vi "MainPicFloatMotV1PIC.vi"() -> ()   [LabVIEW 2010]
uses:
  <vilib>/Instr/_visa.llb/VISA Flush IO Buffer Mask.ctl
  Variable globale 1.vi
  <vilib>/Instr/_visa.llb/VISA Configure Serial Port (Instr).vi
panel:
  out "tableau inversé 2":u8[](array[numeric])
  out "tableau inversé":i8[](array[numeric])
  out "error out 2":errorcluster caption="sortie d'erreur"
  in  "Type":i32=139 min=138 max=139
  out "Float recu":sgl
  in  "Float envoyé":sgl=25.45
  out "Iteration 3":i32
  out "Iteration reception":i32
  out "Iteration Envoi":i32
  out "Checksum calculé":i32
  out "Checksum reçu":i32
  out "Type de donnee (ID)":i32
  out "Byte Start ?":bool
  out "Retour 2":string
  in  "stop secu":bool
  in  "STOP":bool
  out "error out":errorcluster caption="sortie d'erreur"
  in  "baud rate (9600)":u32=9600 caption="débit en bauds (9600)"
  in  "Port Com":refnum<visa-resource-name>="COM7" caption="Nom de ressource VISA"
  # "Envoi"
  # "Réception"
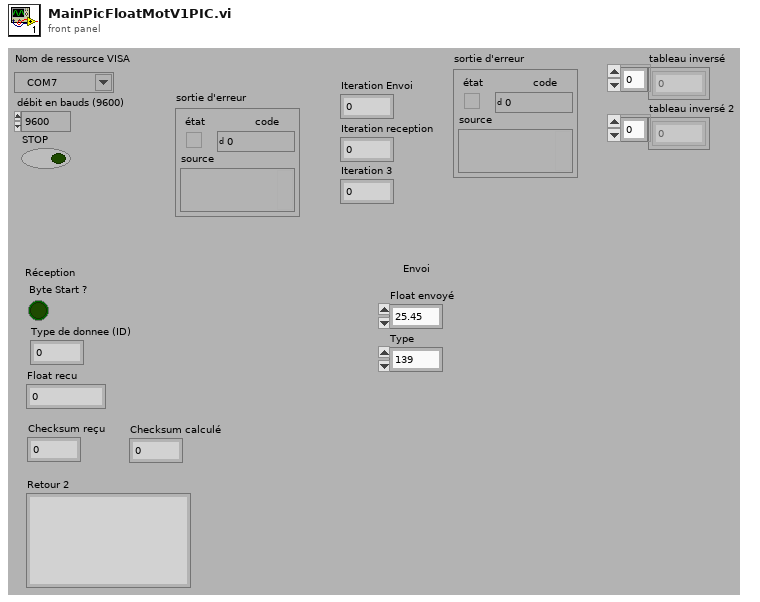
[diagram p1: front panel]
types:
  T1 = typedef "VISA Flush IO Buffer Mask.ctl" = u16
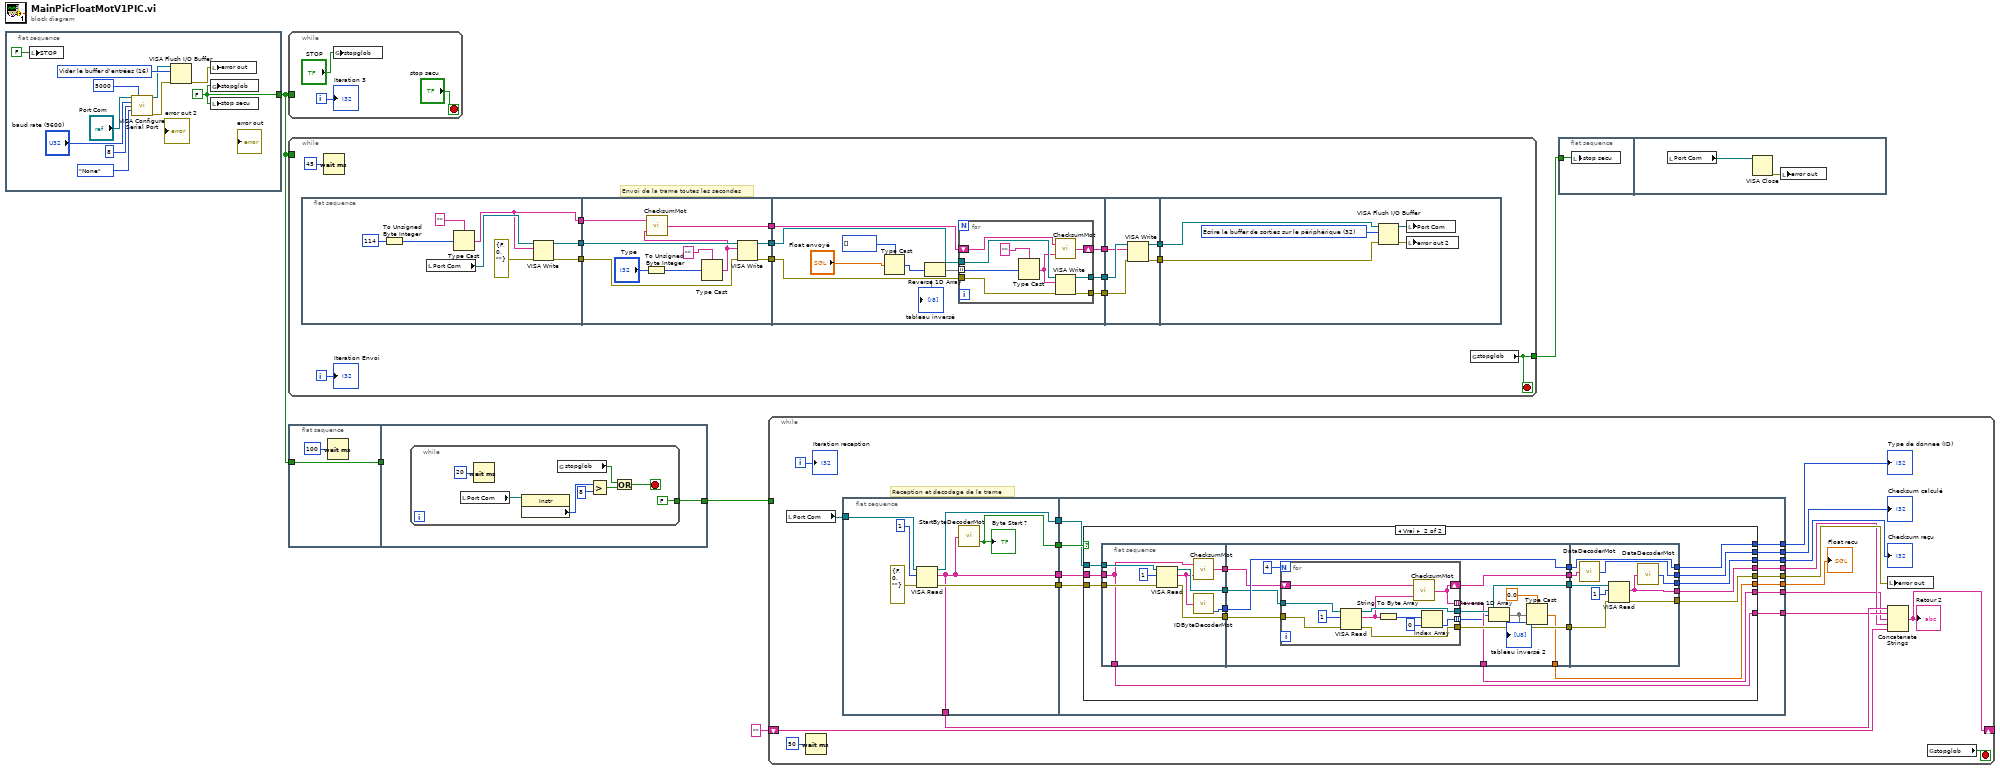
[diagram p0: block diagram]
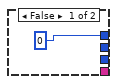
[diagram p2: hidden frame]
diagram:
  n1 = flat-sequence {
    tunnel: [w8] -> w3
    frame #0 {
      w8 = FALSE
      w11 = T1 16 items=["Vider le buffer d'entrées"=16, "Écrire le buffer de sorties sur le périphérique"=32, "Vider le buffer d'entrées (Pas d'E/S)"=64, "Vider le buffer de sorties"=128] ("Mask")
      n2 = local write "STOP"(FALSE) -> ()
      n3 = call-poly "VISA Configure Serial Port"("VISA resource name"="Port Com", "timeout (10sec)"=u32 5000, "baud rate (9600)"="baud rate (9600)", "data bits (8)"=u16 8, "parity (0:none)"=enum16{"None", "Odd", "Even", "Mark", "Space"}."None") -> ("VISA resource name out"=w7:refnum<visa-resource-name>, "error out"=w6:errorcluster)  [unwired: 9 in]
      n4 = VISA Flush I/O Buffer(VISA resource name=w7, mask (16)=w11, error in (no error)=w6) -> (error out=w9:errorcluster)  [unwired: 1 out]
      n5 = local write "error out"(w9) -> ()
      n6 = global write "Variable globale 1.vi" "stopglob"(w8) -> ()
      n7 = local write "stop secu"(w8) -> ()
    }
  }
  n8 = while {
    tunnel: w3 -> [_]
    i -> [w17]
    stop <- "stop secu" stop-if-true
    n9 = global write "Variable globale 1.vi" "stopglob"("STOP") -> ()
    "Iteration 3" <- w17
  }
  n10 = while {
    tunnel: [w27] -> w5
    tunnel: w3 -> [_]
    i -> [w26]
    stop <- w27 stop-if-true
    # "Envoi de la trame toutes les secondes"
    n11 = flat-sequence {
      tunnel: [w38] -> w33
      tunnel: [w37] -> w32
      tunnel: [w36] -> w29
      tunnel: w33 -> [w51]
      tunnel: w32 -> [w50]
      tunnel: [w49] -> w31
      tunnel: [w48] -> w30
      tunnel: w29 -> [w47]
      tunnel: [w46] -> w28
      tunnel: w31 -> [w57]
      tunnel: w30 -> [w59]
      tunnel: w28 -> [w55]
      tunnel: [w58] -> w25
      tunnel: [w56] -> w24
      tunnel: [w54] -> w23
      tunnel: w25 -> [w75]
      tunnel: w24 -> [w74]
      tunnel: w23 -> [w73]
      tunnel: [w72] -> w21
      tunnel: [w71] -> w20
      tunnel: w21 -> [w80]
      tunnel: w20 -> [w79]
      frame #0 {
        n12 = To Unsigned Byte Integer(number=114) -> (unsigned 8bit integer=w35:u8)
        n13 = local read "Port Com"() -> (w41:refnum<visa-resource-name>)
        n14 = Type Cast(type="", x=w35) -> (*(type *) &x=w36:string)
        n15 = VISA Write(VISA resource name=w41, write buffer=w36, error in (no error)=errorcluster {"status"=FALSE, "code"=0, "source"=""} ("entrée d'erreur (pas d'erreur)")) -> (VISA resource name out=w38:refnum<visa-resource-name>, error out=w37:errorcluster)  [unwired: 1 out]
      }
      frame #1 {
        n16 = To Unsigned Byte Integer(number="Type") -> (unsigned 8bit integer=w44:u8)
        n17 = Type Cast(type="", x=w44) -> (*(type *) &x=w42:string)
        n18 = call "ChecksumMot.vi"("Byte2"=w42, "Byte1"=w47) -> ("chaîne"=w46:string)
        n19 = VISA Write(VISA resource name=w51, write buffer=w42, error in (no error)=w50) -> (VISA resource name out=w48:refnum<visa-resource-name>, error out=w49:errorcluster)  [unwired: 1 out]
      }
      frame #2 {
        n20 = Type Cast(type=i8[] [] ("tableau d'octets non signés"), x="Float envoyé") -> (*(type *) &x=w53:i8[])
        n21 = Reverse 1D Array(array=w53) -> (reversed array=w52:i8[])
        "tableau inversé" <- w52
        n22 = for {
          tunnel: w52 -> [w70] mode=indexing
          tunnel: w59 -> [w68]
          tunnel: [w67] -> w58
          tunnel: w57 -> [w66]
          tunnel: [w65] -> w56
          shift-right: [w62] -> w54
          shift-left: w55 -> [w64]
          n23 = Type Cast(type="", x=w70) -> (*(type *) &x=w63:string)
          n24 = call "ChecksumMot.vi"("Byte2"=w63, "Byte1"=w64) -> ("chaîne"=w62:string)
          n25 = VISA Write(VISA resource name=w68, write buffer=w63, error in (no error)=w66) -> (VISA resource name out=w67:refnum<visa-resource-name>, error out=w65:errorcluster)  [unwired: 1 out]
        }
      }
      frame #3 {
        n26 = VISA Write(VISA resource name=w75, write buffer=w73, error in (no error)=w74) -> (VISA resource name out=w72:refnum<visa-resource-name>, error out=w71:errorcluster)  [unwired: 1 out]
      }
      frame #4 {
        w76 = T1 32 items=["Vider le buffer d'entrées"=16, "Écrire le buffer de sorties sur le périphérique"=32, "Vider le buffer d'entrées (Pas d'E/S)"=64, "Vider le buffer de sorties"=128] ("Mask")
        n27 = VISA Flush I/O Buffer(VISA resource name=w80, mask (16)=w76, error in (no error)=w79) -> (VISA resource name out=w77:refnum<visa-resource-name>, error out=w78:errorcluster)
        n28 = local write "Port Com"(w77) -> ()
        n29 = local write "error out 2"(w78) -> ()
      }
    }
    n30 = Wait (ms)(milliseconds to wait=u32 45 ("attente (ms)")) -> ()  [unwired: 1 out]
    n31 = global read "Variable globale 1.vi" "stopglob"() -> (w27:bool)
    "Iteration Envoi" <- w26
  }
  n32 = flat-sequence {
    tunnel: w3 -> [w81]
    tunnel: [w81] -> w2
    tunnel: w2 -> [_]
    tunnel: [w83] -> w1
    frame #0 {
      n33 = Wait (ms)(milliseconds to wait=u32 100 ("attente (ms)")) -> ()  [unwired: 1 out]
    }
    frame #1 {
      n34 = while {
        tunnel: [FALSE] -> w83
        stop <- w90 stop-if-true
        n35 = local read "Port Com"() -> (w89:refnum<visa-resource-name>)
        n36 = Wait (ms)(milliseconds to wait=u32 20 ("attente (ms)")) -> ()  [unwired: 1 out]
        n37 = property class="Instr"(reference=w89) -> ("Serial Settings:Number of Bytes at Serial Port"=w88:u32)  [unwired: 1 in, 2 out]
        n38 = global read "Variable globale 1.vi" "stopglob"() -> (w91:bool)
        n39 = Greater?(x=w88, y=u32 8) -> (0:w86:bool)
        n40 = Or(x=w91, y=w86) -> (x .or. y?=w90:bool)
      }
    }
  }
  n41 = while {
    shift-right: [w95] -> _
    shift-left: "" -> [w96]
    tunnel: w1 -> [_]
    i -> [w94]
    stop <- w110 stop-if-true
    # "Reception et decodage de la trame"
    n42 = local read "Port Com"() -> (w108:refnum<visa-resource-name>)
    n43 = Wait (ms)(milliseconds to wait=u32 50 ("attente (ms)")) -> ()  [unwired: 1 out]
    n44 = flat-sequence {
      tunnel: w108 -> [w116]
      tunnel: [w115] -> w107
      tunnel: [w114] -> w106
      tunnel: [w113] -> w105
      tunnel: [w112] -> w103
      tunnel: [w112] -> w99
      tunnel: w107 -> [w129]
      tunnel: w106 -> [w128]
      tunnel: w105 -> [w127]
      tunnel: [w126] -> w104
      tunnel: w103 -> [w125]
      tunnel: [w124] -> w102
      tunnel: [w123] -> w101
      tunnel: [w122] -> w100
      tunnel: [w121] -> w98
      tunnel: [w120] -> w97
      tunnel: [w119] -> w93
      tunnel: [w118] -> w92
      frame #0 {
        n45 = VISA Read(VISA resource name=w116, byte count=u32 1 ("nombre d'octets"), error in (no error)=errorcluster {"status"=FALSE, "code"=0, "source"=""} ("entrée d'erreur (pas d'erreur)")) -> (VISA resource name out=w114:refnum<visa-resource-name>, read buffer=w112:string, error out=w113:errorcluster)  [unwired: 1 out]
        n46 = call "StartByteDecoderMot.vi"("byte1"=w112) -> ("Byte Start ?"=w115:bool)  [unwired: 1 in]
        "Byte Start ?" <- w115
      }
      frame #1 {
        n47 = case shown="Vrai" w129 {
          tunnel: w128 -> [_ w149]
          tunnel: w127 -> [_ w148]
          tunnel: [0 ("Type de donnee (ID)") w147] -> w126
          tunnel: w125 -> [_ w142]
          tunnel: [_ w140] -> w124
          tunnel: [_ w139] -> w123
          tunnel: [_ w138] -> w122
          tunnel: [_ w137] -> w121
          tunnel: [_ w136] -> w120
          tunnel: [_ w133] -> w119
          tunnel: [_ w131] -> w118
          frame False {
          }
          frame True {
            n48 = flat-sequence {
              tunnel: w149 -> [w158]
              tunnel: w148 -> [w157]
              tunnel: [w155] -> w146
              tunnel: [w154] -> w145
              tunnel: [w153] -> w144
              tunnel: w142 -> [w150]
              tunnel: [w151] -> w141
              tunnel: [w150] -> w137
              tunnel: w146 -> [w171]
              tunnel: w145 -> [w170]
              tunnel: w144 -> [w167]
              tunnel: [w171] -> w143
              tunnel: w141 -> [w164]
              tunnel: [w169] -> w135
              tunnel: [w168] -> w134
              tunnel: [w165] -> w133
              tunnel: [w163] -> w132
              tunnel: [w161] -> w131
              tunnel: [w191] -> w147
              tunnel: w143 -> [w191]
              tunnel: [w189] -> w140
              tunnel: [w188] -> w139
              tunnel: [w187] -> w138
              tunnel: [w186] -> w136
              tunnel: w135 -> [w185]
              tunnel: w134 -> [w184]
              tunnel: w132 -> [w183]
              frame #0 {
                n49 = VISA Read(VISA resource name=w158, byte count=u32 1 ("nombre d'octets"), error in (no error)=w157) -> (VISA resource name out=w154:refnum<visa-resource-name>, read buffer=w152:string, error out=w153:errorcluster)  [unwired: 1 out]
                n50 = call "ChecksumMot.vi"("Byte2"=w152, "Byte1"=w150) -> ("chaîne"=w151:string)
                n51 = call "IDByteDecoderMot.vi"("byte1"=w152) -> ("Type de donnee (ID)"=w155:i32)  [unwired: 2 out]
              }
              frame #1 {
                n52 = for {
                  N: 4 -> [_]
                  tunnel: w170 -> [w181]
                  tunnel: [w180] -> w169
                  tunnel: [w179] -> w168
                  tunnel: w167 -> [w178]
                  tunnel: [w175] -> w160 mode=indexing
                  shift-right: [w172] -> w163
                  shift-left: w164 -> [w174]
                  tunnel: [w172] -> w161 mode=indexing
                  n53 = VISA Read(VISA resource name=w181, byte count=u32 1 ("nombre d'octets"), error in (no error)=w178) -> (VISA resource name out=w180:refnum<visa-resource-name>, read buffer=w173:string, error out=w179:errorcluster)  [unwired: 1 out]
                  n54 = String To Byte Array(string=w173) -> (unsigned byte array=w177:u8[])
                  n55 = call "ChecksumMot.vi"("Byte2"=w173, "Byte1"=w174) -> ("chaîne"=w172:string)
                  n56 = Index Array(array=w177, index=0 ("indice")) -> (element=w175:u8)
                }
                n57 = Reverse 1D Array(array=w160) -> (reversed array=w159:u8[])
                "tableau inversé 2" <- w159
                n58 = Type Cast(type=sgl 0.0, x=w159) -> (*(type *) &x=w165:sgl)
              }
              frame #2 {
                n59 = call "DataDecoderMot.vi"("byte1"=w183) -> ("Data"=w189:i32)
                n60 = VISA Read(VISA resource name=w185, byte count=u32 1 ("nombre d'octets"), error in (no error)=w184) -> (read buffer=w186:string, error out=w187:errorcluster)  [unwired: 2 out]
                n61 = call "DataDecoderMot.vi"("byte1"=w186) -> ("Data"=w188:i32)
              }
            }
          }
        }
      }
    }
    n62 = local write "error out"(w100) -> ()
    n63 = Concatenate Strings(w99, w98, w92, w97, w96) -> (w95:string)
    "Retour 2" <- w95
    n64 = global read "Variable globale 1.vi" "stopglob"() -> (w110:bool)
    "Type de donnee (ID)" <- w104
    "Checksum reçu" <- w101
    "Checksum calculé" <- w102
    "Iteration reception" <- w94
    "Float recu" <- w93
  }
  n65 = flat-sequence {
    tunnel: w5 -> [w192]
    frame #0 {
      n66 = local write "stop secu"(w192) -> ()
    }
    frame #1 {
      n67 = local read "Port Com"() -> (w194:refnum<visa-resource-name>)
      n68 = VISA Close(VISA resource name=w194) -> (error out=w193:errorcluster)  [unwired: 1 in]
      n69 = local write "error out"(w193) -> ()
    }
  }
